vi "Do Core.vi"(8 "error in (no error)":errorcluster, 9 "Actor in":refnum<class "Actor.lvclass">, 11 "Reply Message":refnum<class "GetReceiveDataBuffer Msg.lvclass">) -> (0 "error out":errorcluster, 1 "Actor out":refnum<class "Actor.lvclass">, 2 "Reply":variant)   [LabVIEW 2022 SP3, in "TcpServer.lvlib" / "GetReceiveDataBuffer Msg.lvclass"]
doc: "(<B>Filename</B>: Actor Framework.lvlib:Reply Msg.lvclass:Do Core.vi)\n\nDefines what an actor does when it receives <B>Reply Message</B>. This method also defines the <B>Reply</B> that is returned to the actor that sent <B>Reply Message</B>.\n\nBy default, this method does nothing, and <B>Reply</B> is the ancestor Message class. A child class must override this method to define behavior and specify a child of the Message class to return in the <B>Reply</B> output."
uses:
  GetReceiveDataBuffer Msg.lvclass
  GetReceiveDataBuffer Msg.lvclass/GetReceiveDataBuffer Msg.ctl
  1042b927-0ffd-4c8c-b955-fb69b4dea291.vi
  TcpServer/TcpServer.lvclass
  <vilib>/ActorFramework/Actor/Actor.lvclass
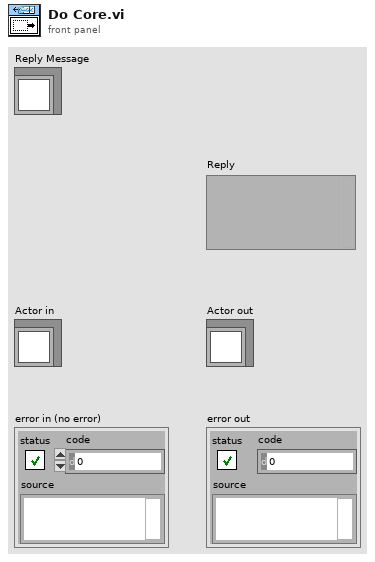
[diagram p1: front panel]
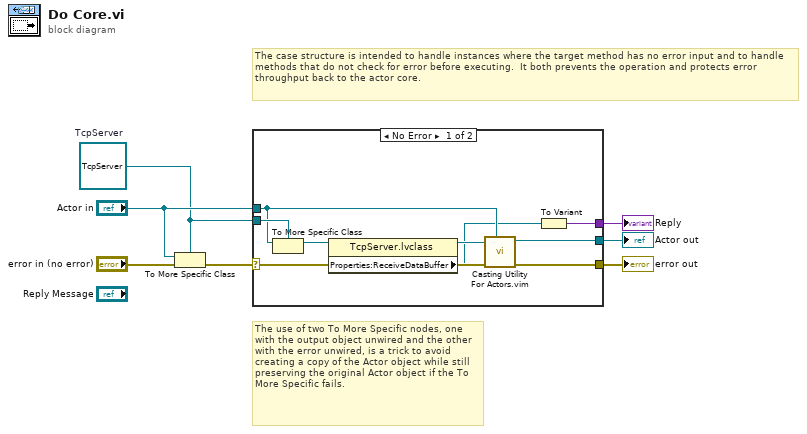
[diagram p0: block diagram]
diagram:
  w4 = refnum<class "TcpServer.lvclass"> refnum  # TcpServer
  # "The use of two To More Specific nodes, one with the output object unwired and the other with the error unwired, is a trick to avoid creating a copy of the Actor object while still preserving the original Actor object if the To More Specific fails."
  # "The case structure is intended to handle instances where the target method has no error input and to handle methods that do not check for error before executing.  It both prevents the operation and protects error throughput back to the actor core."
  n1 = To More Specific Class(target class=w4, reference="Actor in", error in="error in (no error)") -> (error out=w7:errorcluster)  [unwired: 1 out]
  n2 = case shown="No Error" w7 {
    selector: w7 -> [w16 w18]
    tunnel: [w12 w18] -> w3
    tunnel: [w13 w17] -> w2
    tunnel: "Actor in" -> [w14 w17]
    tunnel: w4 -> [w15 _]
    tunnel: [w10 _] -> w1
    frame No Error {
      n3 = To More Specific Class(target class=w15, reference=w14) -> (specific class reference=w11:refnum<class "TcpServer.lvclass">)  [unwired: 1 in, 1 out]
      n4 = property class="TcpServer.lvclass"(reference=w11) -> (reference out=w9:refnum<class "TcpServer.lvclass">, "Properties:ReceiveDataBuffer"=w8:refnum<queue>)  [unwired: 1 in, 1 out]
      n5 = call "Casting Utility For Actors.vim"("type"=w14, "error in (no error)"=w16, "Actor in"=w9) -> ("error out"=w12:errorcluster, "Actor out"=w13:refnum<class "Actor.lvclass">)  [unwired: 7 in]
      n6 = To Variant(anything=w8) -> (Variant=w10:variant)
    }
    frame Error {
      # "If type check fails, pass the original object out again."
    }
  }
  "error out" <- w3
  "Actor out" <- w2
  "Reply" <- w1
